vi "JSON Generator.vi"(8 "error in (no error)":errorcluster, 9 "ECU":refnum<k21>="GIP\ncan_messages_818", 10 "XNET Database":refnum<k21>="GIP_CAN_Database", 11 "CAN in":refnum<class "CAN.lvclass">) -> (0 "error out":errorcluster, 3 "CAN out":refnum<class "CAN.lvclass">)   [LabVIEW 2019, in "CAN.lvclass"]
uses:
  CAN.lvclass
  CAN.lvclass/CAN.ctl
  <vilib>/JDP Science/JSONtext/Get all Object Items.vi
  <vilib>/JDP Science/JSONtext/Set Multiple Object Items.vi
  <resource>/objmgr/xnet.rc
  <vilib>/JDP Science/JSONtext/JSONtext.lvlib
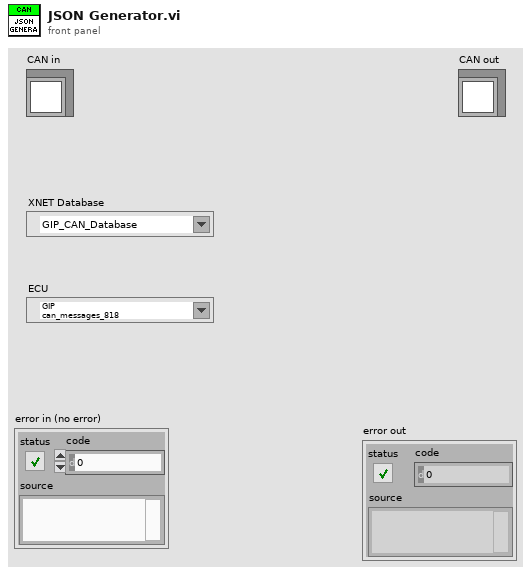
[diagram p1: front panel]
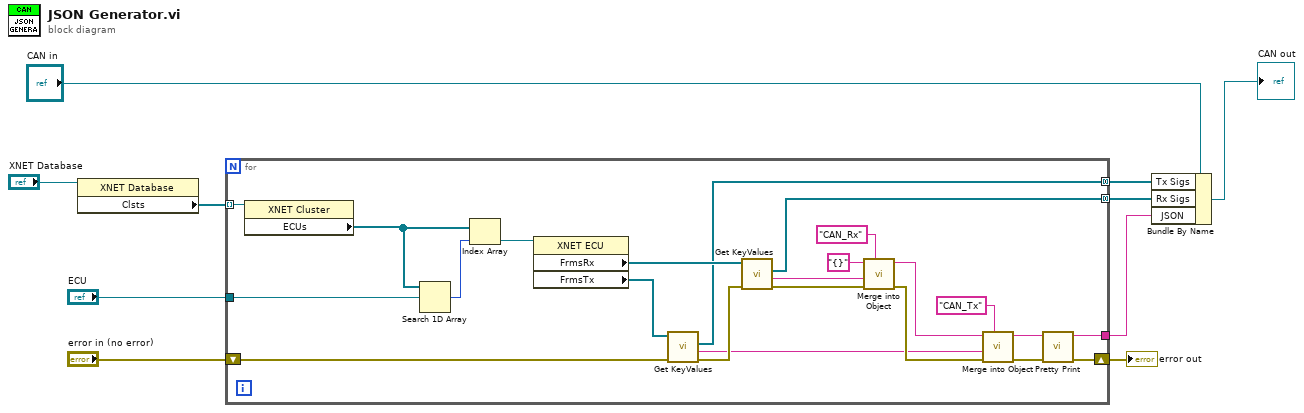
[diagram p0: block diagram]
diagram:
  n1 = property class="XNET Database"(reference="XNET Database") -> ("Clsts"=w9:refnum<k21>[])  [unwired: 1 in, 2 out]
  n2 = for {
    tunnel: w9 -> [w18] mode=indexing
    shift-right: [w28] -> w7
    shift-left: "error in (no error)" -> [w31]
    tunnel: [w11] -> w1
    tunnel: "ECU" -> [w16]
    tunnel: [w13] -> w3 mode=concatenating
    tunnel: [w12] -> w2 mode=concatenating
    n3 = property class="XNET Cluster"(reference=w18) -> ("ECUs"=w17:refnum<k21>[])  [unwired: 1 in, 2 out]
    n4 = Search 1D Array(1D array=w17, element=w16) -> (index of element=w33:i32)  [unwired: 1 in]
    n5 = Index Array(array=w17, index=w33) -> (element=w32:refnum<k21>)
    n6 = property class="XNET ECU"(reference=w32) -> ("FrmsRx"=w15:refnum<k21>[], "FrmsTx"=w14:refnum<k21>[])  [unwired: 1 in, 2 out]
    n7 = call "Get KeyValues.vi"("error in (no error)"=w31, "Frames"=w14) -> ("error out"=w27:errorcluster, "<JSON>"=w20:string, "Sigs"=w13:refnum<k21>[])  [unwired: 6 in, 1 out]
    n8 = call "Get KeyValues.vi"("error in (no error)"=w27, "Frames"=w15) -> ("error out"=w26:errorcluster, "<JSON>"=w19:string, "Sigs"=w12:refnum<k21>[])  [unwired: 6 in, 1 out]
    n9 = call <vilib>:"Merge into Object.vi"("$Path or Item Name"="CAN_Rx", "error in (no error)"=w26, "JSON Object to Merge"=w19, "JSON"="{}") -> ("error out"=w24:errorcluster, "<JSON>"=w23:string)  [unwired: 5 in]
    n10 = call <vilib>:"Merge into Object.vi"("$Path or Item Name"="CAN_Tx", "error in (no error)"=w24, "JSON Object to Merge"=w20, "JSON"=w23) -> ("error out"=w30:errorcluster, "<JSON>"=w29:string)  [unwired: 5 in]
    n11 = call <vilib>:"Pretty Print.vi"("error in (no error)"=w30, "JSON"=w29) -> ("error out"=w28:errorcluster, "<JSON>"=w11:string)  [unwired: 7 in, 1 out]
  }
  "error out" <- w7
  n12 = Bundle By Name(cluster="CAN in", "Tx Sigs"=w3, "Rx Sigs"=w2, "JSON"=w1) -> (→"CAN out":refnum<class "CAN.lvclass">)
